vi "connect PG server.vi"(8 "error in (no error)":errorcluster, 11 "SP in":refnum<class "PG alarms.lvclass">) -> (0 "error out":errorcluster, 2 "conn_out":u64, 3 "SP out":refnum<class "PG alarms.lvclass">)   [LabVIEW 2019, in "PG alarms.lvclass"]
uses:
  PG alarms.lvclass
  C:/my_projects/projects/Algorithms/Labview/19/Database/Save messages PGserver/Save messages PGserver.lvclass
  Save messages PGserver/Save messages PGserver.lvclass/Save messages PGserver.ctl
  PostgreSQL2LabVIEW/libpqlv64/src/PQfinish.vi
  PostgreSQL2LabVIEW/libpqlv64/src/PQconnectdb.vi
  PostgreSQL2LabVIEW/libpqlv64/src/PQerrorMessage.vi
  PostgreSQL2LabVIEW/libpqlv64/src/PQstatus.vi
  <vilib>/dlg_ctls.llb/Space Constant.vi
  PostgreSQL2LabVIEW/libpqUtility64/src/PQexecute.vi
  PostgreSQL2LabVIEW/libpqUtility64/src/PQlistSequenses.vi
  PostgreSQL2LabVIEW/libpqlv64/src/PQresultErrorMessage.vi
  PostgreSQL2LabVIEW/libpqUtility64/src/PQclear.vi
  PostgreSQL2LabVIEW/libpqlv64/src/PQsendQuery.vi
  PostgreSQL2LabVIEW/libpqlv64/src/PQgetResult.vi
  PostgreSQL2LabVIEW/libpqlv64/src/PQresultStatus.vi
  PostgreSQL2LabVIEW/libpqUtility64/src/PQgetColumn.vi
  PostgreSQL2LabVIEW/libpqlv64/src/PQclear.vi
  PostgreSQL2LabVIEW/libpqUtility64/src/PQfetchTables.vi
  PostgreSQL2LabVIEW/libpqlv64/src/PQgetvalue.vi
  PostgreSQL2LabVIEW/libpqlv64/src/PQntuples.vi
  PostgreSQL2LabVIEW/libpqUtility64/libpqutility64.lvlib
  PostgreSQL.lvlib
  Save messages PGserver/Save messages PGserver.lvclass
panel:
  out "PQStatus":T1(ring)
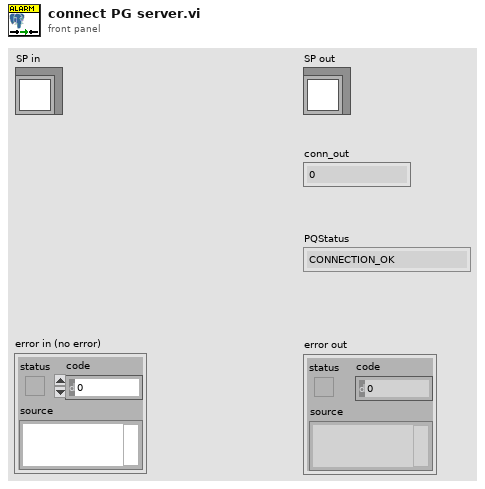
[diagram p1: front panel]
types:
  T1 = enum32{"CONNECTION_OK", "CONNECTION_BAD", "CONNECTION_STARTED", "CONNECTION_MADE", "CONNECTION_AWAITING_RESPONSE", "CONNECTION_AUTH_OK", "CONNECTION_SETENV", "CONNECTION_SSL_STARTUP", "CONNECTION_NEEDED"}
  T2 = typedef "PostgreSQL.lvlib/Coninfo.ctl" = cluster{"host":string, "port":string, "client_encoding":string, "dbname":string, "user":string, "password":string}
  T3 = cluster{"table postfix":string, "sequence name":string, "columns name":string[], "columns type":string}
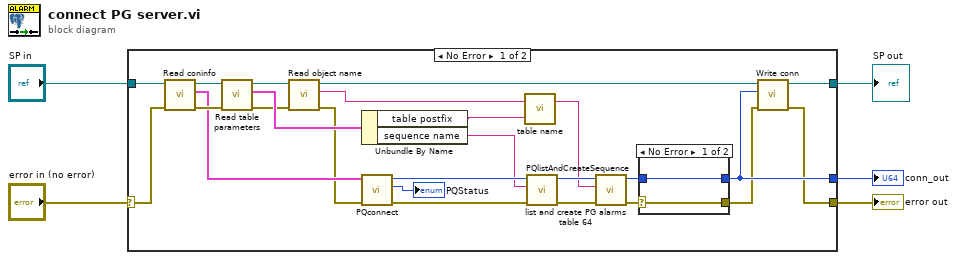
[diagram p0: block diagram]
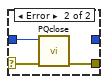
[diagram p2: hidden frame]
diagram:
  n1 = case shown="No Error" "error in (no error)" {
    selector: "error in (no error)" -> [w18 w36]
    tunnel: [w14 w36] -> w4
    tunnel: [w16 w37] -> w2
    tunnel: "SP in" -> [w22 w37]
    tunnel: [w17 _] -> w1
    frame No Error {
      n2 = call "Read coninfo.vi"("error in (no error)"=w18, "SP in"=w22) -> ("error out"=w21:errorcluster, "conninfo"=w19:T2, "SP out"=w20:refnum<class "PG alarms.lvclass">)  [unwired: 7 in]
      n3 = call "Read table parameters.vi"("error in (no error)"=w21, "SP in"=w20) -> ("error out"=w9:errorcluster, "table parameters"=w13:T3, "SP out"=w10:refnum<class "PG alarms.lvclass">)  [unwired: 7 in]
      n4 = call "Read object name.vi"("error in (no error)"=w9, "SP in"=w10) -> ("error out"=w8:errorcluster, "object name"=w7:string, "SP out"=w6:refnum<class "PG alarms.lvclass">)  [unwired: 7 in]
      n5 = Unbundle By Name(w13) -> ("table postfix"=w12:string, "sequence name"=w11:string)
      n6 = call "PQconnect.vi"("error in (no error)"=w8, "conninfo"=w19) -> ("error out"=w29:errorcluster, "PQStatus"=→"PQStatus":T1, "conn"=w27:u64)  [unwired: 7 in]
      n7 = call "table name.vi"("postfix"=w12, "object name"=w7) -> ("table name"=w23:string)  [unwired: 1 in]
      n8 = call "PQlistAndCreateSequence.vi"("error in"=w29, "sequence name"=w11, "conn"=w27) -> ("error out"=w30:errorcluster, "conn_out"=w28:u64)  [unwired: 7 in]
      n9 = call "list and create PG alarms table 64.vi"("error in"=w30, "table name"=w23, "conn"=w28) -> ("error out"=w26:errorcluster, "conn_out"=w25:u64)  [unwired: 7 in]
      n10 = case shown="No Error" w26 {
        selector: w26 -> [w31 w34]
        tunnel: w25 -> [w32 w35]
        tunnel: [w32 _] -> w17
        tunnel: [w31 w33] -> w15
        frame No Error {
        }
        frame Error {
          n11 = call "PQclose.vi"("error in (no error)"=w34, "conn"=w35) -> ("error out"=w33:errorcluster)  [unwired: 9 in]
        }
      }
      n12 = call "Write conn.vi"("error in (no error)"=w15, "conn"=w17, "SP in"=w6) -> ("error out"=w14:errorcluster, "SP out"=w16:refnum<class "PG alarms.lvclass">)  [unwired: 7 in]
    }
    frame Error {
    }
  }
  "error out" <- w4
  "SP out" <- w2
  "conn_out" <- w1
